vi "OptionSelect3.vi"() -> ()   [LabVIEW 2015]
panel:
  in  "stop":bool
  out "element":T1(ring)
  out "index of element":i32
  out "appended array":bool[](array[boolean])
  in  "$50":bool
  in  "$20":bool
  in  "$10":bool
  in  "$5":bool
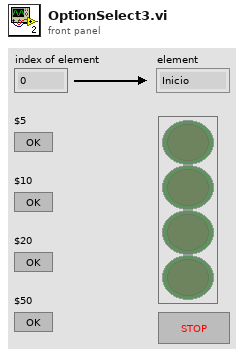
[diagram p1: front panel]
types:
  T1 = enum16{"Inicio", "En espera", "$5", "$10", "$20", "$50", "Cambiar", "Producto", "Salir"}
  T2 = enum16{"Inicio", "En espera", "$5", "$10", "$20", "$50", "Cambiar", "Producto", "Salir"}[]
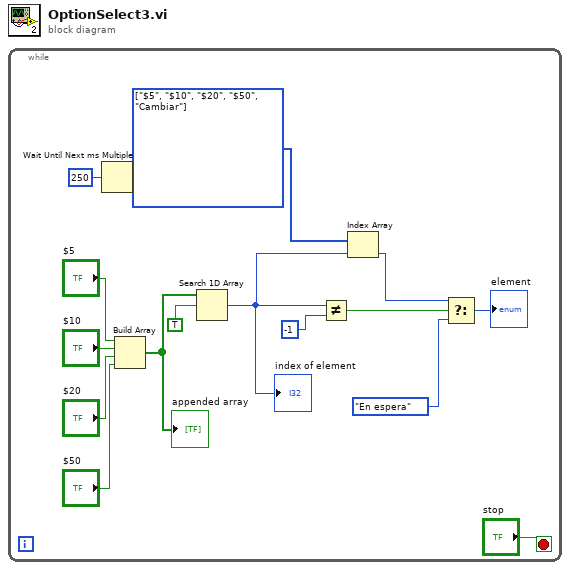
[diagram p0: block diagram]
diagram:
  n1 = while {
    stop <- "stop" stop-if-true
    w7 = T2 [enum."$5", enum."$10", enum."$20", enum."$50", enum."Cambiar"] items=["Inicio", "En espera", "$5", "$10", "$20", "$50", "Cambiar", "Producto", "Salir"]
    n2 = Wait Until Next ms Multiple(millisecond multiple=u32 250) -> ()  [unwired: 1 out]
    n3 = Build Array("$5", "$10", "$20", "$50") -> (w11:bool[])
    "appended array" <- w11
    n4 = Search 1D Array(1D array=w11, element=TRUE) -> (index of element=w6:i32)  [unwired: 1 in]
    "index of element" <- w6
    n5 = Not Equal?(x=w6, y=-1) -> (x != y?=w5:bool)
    n6 = Index Array(array=w7, index=w6) -> (element=w4:T1)
    n7 = Select(t=w4, s=w5, f=T1."En espera") -> (s? t:f=→"element":T1)
  }
